vi "circ_ap && lens && forvard.vi"() -> ()   [LabVIEW 2012, in "LightPipes.lvlib"]
uses:
  LightPipes.lvlib
panel:
  out "Field":cluster{"n_grid":i32, "size":dbl, "lambda":dbl}
  # "Beam"
  # "Circula Apparature"
  # "Lens"
  # "Forvard"
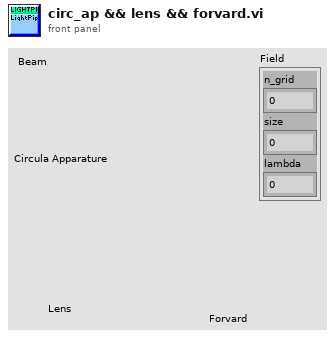
[diagram p1: front panel]
types:
  T1 = cluster{"n_grid":i32, "@dummy control@":i8, "@dummy control@":i8, "@dummy control@":i8, "@dummy control@":i8, "size":dbl, "lambda":dbl, "int1":i32, "int2":i32, "int3":i32, "@dummy control@":i8, "@dummy control@":i8, "@dummy control@":i8, "@dummy control@":i8, "double1":dbl, "double2":dbl, "double3":dbl, "real":u32, "imaginary":u32}
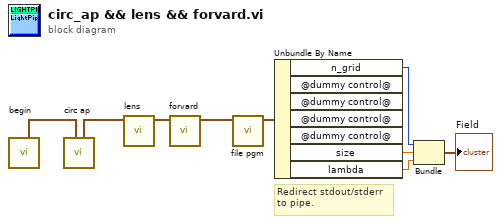
[diagram p0: block diagram]
diagram:
  # "Redirect stdout/stderr\nto pipe."
  n1 = call "begin.vi"() -> ("field out"=w6:T1)  [unwired: 11 in]
  n2 = call "circ ap.vi"("field"=w6) -> ("field out"=w5:T1)  [unwired: 10 in]
  n3 = call "lens.vi"("field"=w5) -> ("field out"=w4:T1)  [unwired: 10 in]
  n4 = call "forvard.vi"("field"=w4) -> ("field out"=w3:T1)  [unwired: 10 in]
  n5 = call "file pgm.vi"("field"=w3) -> ("field out"=w2:T1)  [unwired: 9 in, 1 out]
  n6 = Unbundle By Name(w2) -> ("n_grid"=w7:i32, "size"=w8:dbl, "lambda"=w9:dbl)  [unwired: 4 out]
  n7 = Bundle("n_grid"=w7, "size"=w8, "lambda"=w9) -> (→"Field":cluster{"n_grid":i32, "size":dbl, "lambda":dbl})  [unwired: 1 in]
